vi "Set Process State.vi"(8 "error in (no error)":errorcluster, 9 "Payload":variant, 10 "Command":string, 11 "Process in":refnum<class "Process.lvclass">) -> (0 "error out":errorcluster, 3 "Process out":refnum<class "Process.lvclass">)   [LabVIEW 2019, in "TimingDRV Engine.lvlib" / "Process.lvclass"]
uses:
  Process.lvclass
  TypeDefs/Message.ctl
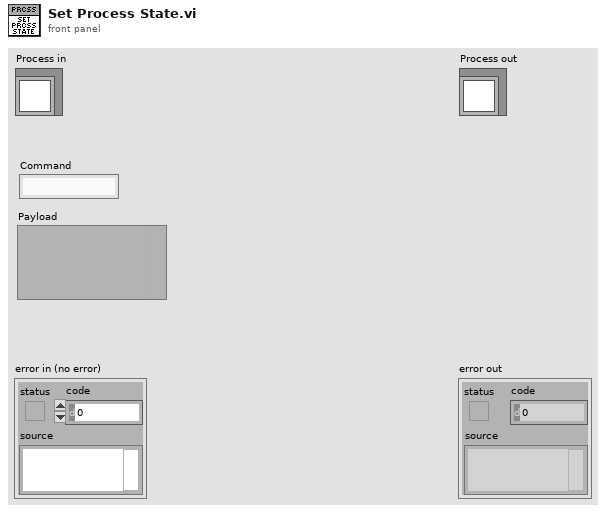
[diagram p1: front panel]
types:
  T1 = typedef "TimingDRV Engine.lvlib/Process.lvclass/Message.ctl" = cluster{"Command":string, "Payload":variant}
  T2 = typedef "TimingDRV Engine.lvlib/Process.lvclass/Process Lookup.ctl" = cluster{"Process ID":string, "MessageQ":refnum<queue>, "Update UE":refnum<user-event>}
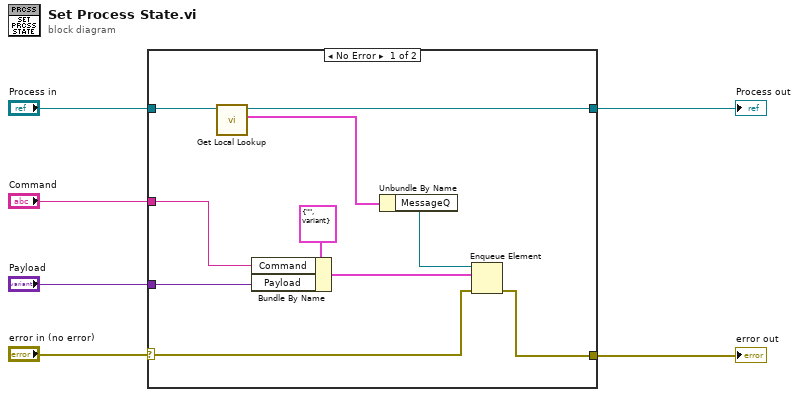
[diagram p0: block diagram]
diagram:
  n1 = case shown="No Error" "error in (no error)" {
    selector: "error in (no error)" -> [w8 w18]
    tunnel: [w15 w18] -> w5
    tunnel: [w7 w17] -> w3
    tunnel: "Process in" -> [w13 w17]
    tunnel: "Command" -> [w10 _]
    tunnel: "Payload" -> [w9 _]
    frame No Error {
      n2 = call-dynamic "Get Local Lookup.vi"("Process in"=w13) -> ("Process Lookup"=w16:T2, "Process out"=w7:refnum<class "Process.lvclass">)  [unwired: 8 in, 1 out]
      n3 = Bundle By Name(cluster=T1 {"Command"="", "Payload"=variant} ("element"), "Command"=w10, "Payload"=w9) -> (w11:T1)
      n4 = Unbundle By Name(w16) -> ("MessageQ"=w14:refnum<queue>)
      n5 = Enqueue Element(queue=w14, element=w11, error in (no error)=w8) -> (error out=w15:errorcluster)  [unwired: 1 in, 2 out]
    }
    frame Error {
    }
  }
  "error out" <- w5
  "Process out" <- w3
